vi "温度设置.vi"() -> ()   [LabVIEW 2015]
uses:
  <vilib>/Utility/file.llb/Write Delimited Spreadsheet (string).vi
  <vilib>/Utility/file.llb/Read Delimited Spreadsheet (string).vi
panel:
  in  "载入":bool
  in  "表格":string[][](table)
  in  "保存编号":bool
  in  "清空编号":bool
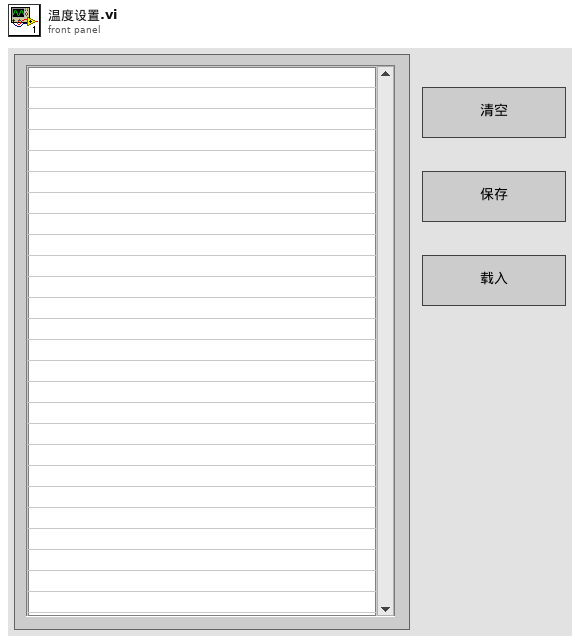
[diagram p1: front panel]
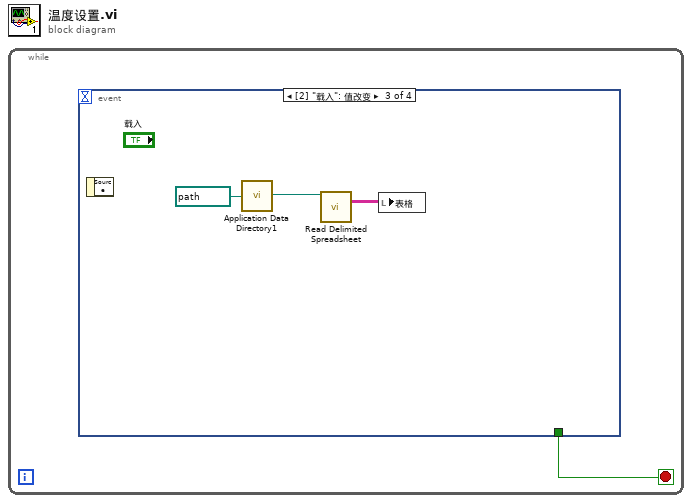
[diagram p0: block diagram]
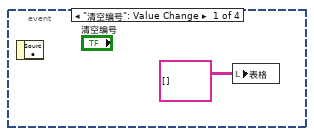
[diagram p2: hidden frame]
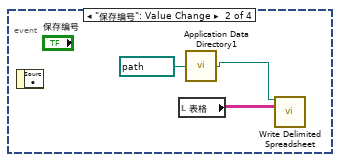
[diagram p3: hidden frame]
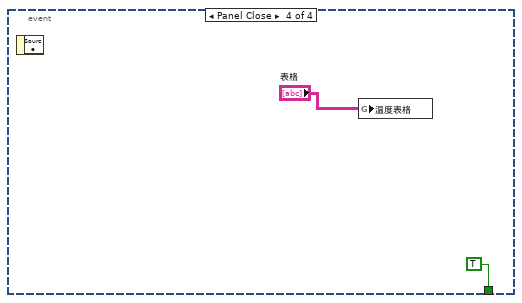
[diagram p4: hidden frame]
diagram:
  n1 = while {
    stop <- w1 stop-if-true
    n2 = event shown="[2] \"载入\": 值改变" {
      selector: _ -> [_ _ _ _]
      dyn-events: _ -> [_ _ _ _]
      timeout: _ -> [_ _ _ _]
      tunnel: [_ _ _ TRUE] -> w1
      event "清空编号": Value Change {
        n3 = event-data() -> ()  [unwired: 1 in, 1 out]
        n4 = local write "表格"(string[][] [] ("项名")) -> ()
      }
      event "保存编号": Value Change {
        n5 = event-data() -> ()  [unwired: 1 in, 1 out]
        n6 = local read "表格"() -> (w5:string[][])
        n7 = call "Application Data Directory1.vi"("Relative path (.)"=path "温度.txt") -> ("Application Directory (+ Relative)"=w3:path)
        n8 = call-poly <vilib>:"Write Delimited Spreadsheet.vi"("file path (dialog if empty)"=w3, "2D data"=w5) -> ()  [unwired: 12 in, 2 out]
      }
      event "载入": Value Change {
        n9 = event-data() -> ()  [unwired: 1 in, 1 out]
        n10 = call "Application Data Directory1.vi"("Relative path (.)"=path "温度.txt") -> ("Application Directory (+ Relative)"=w6:path)
        n11 = call-poly <vilib>:"Read Delimited Spreadsheet.vi"("file path (dialog if empty)"=w6) -> ("all rows"=w8:string[][])  [unwired: 9 in, 5 out]
        n12 = local write "表格"(w8) -> ()
      }
      event Panel Close {
        n13 = event-data() -> ()  [unwired: 1 in, 1 out]
        n14 = global write "全局.vi" "温度表格"("表格") -> ()
      }
    }
  }
